vi "projet.vi"() -> ()   [LabVIEW 2020]
panel:
  out "message":string
  out "etage":i32
  out "A":bool
  out "E3":bool
  in  "C_3":bool
  in  "C_ 2":bool
  in  "C_1":bool
  in  "C_0":bool
  in  "3 Button":bool
  in  "2 Button":bool
  in  "1 Button":bool
  in  "0 Button":bool
  out "RDC":bool
  out "E1":bool
  out "E2":bool
  # "dans ce  projet :\nona 5 evenements :\n              -wait for postion (l'attente pour cliquer sur les buttons)\n             - le clique sur le button 0  (appel de l'ascenseur au RDC)\n              - le clique sur le button 1 (appel de l'ascenseur au  1ère étage)\n               -le clique sur le button 2  (appel de l'ascenseur au  2ème étage)\n              - le clique sur le button 3 (appel de l'ascenseur au  3ème étage)\n-un message  pour expliquer  la 1er etape de demarage de ce projet \n-chaque transition d' un etage à un  autre  se fait par le clique sur les capteur indiquant\nl'étage actuel et afficher son numéro dans l 'indicateur  \"etage\"\n-led A  : \"open\" lorsque  ona arrivee   à la destination \nona fait la comparison avec les button de capteur   dans chaque evenement \npar exemple  lorsque ona clique sur le button1 on peut trouver dans C-3 ,C-2,C-1,C-0\net la clique   sur le capteur C-3 va desactiver les capteur C-0 , C-1 et l' atttente pour cliquer\nsur le capteur C-2 , ce clique permet d'activer C-1et desactiverC-3  ect ..."
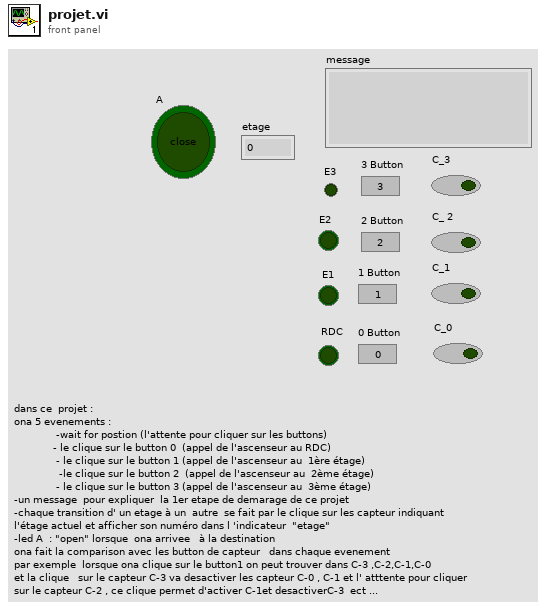
[diagram p1: front panel]
types:
  T1 = enum16{"wait for postion", "B1", "B2", "B3", "B0"}
  T2 = enum8{"Enabled", "Disabled", "Disabled and Grayed Out"}
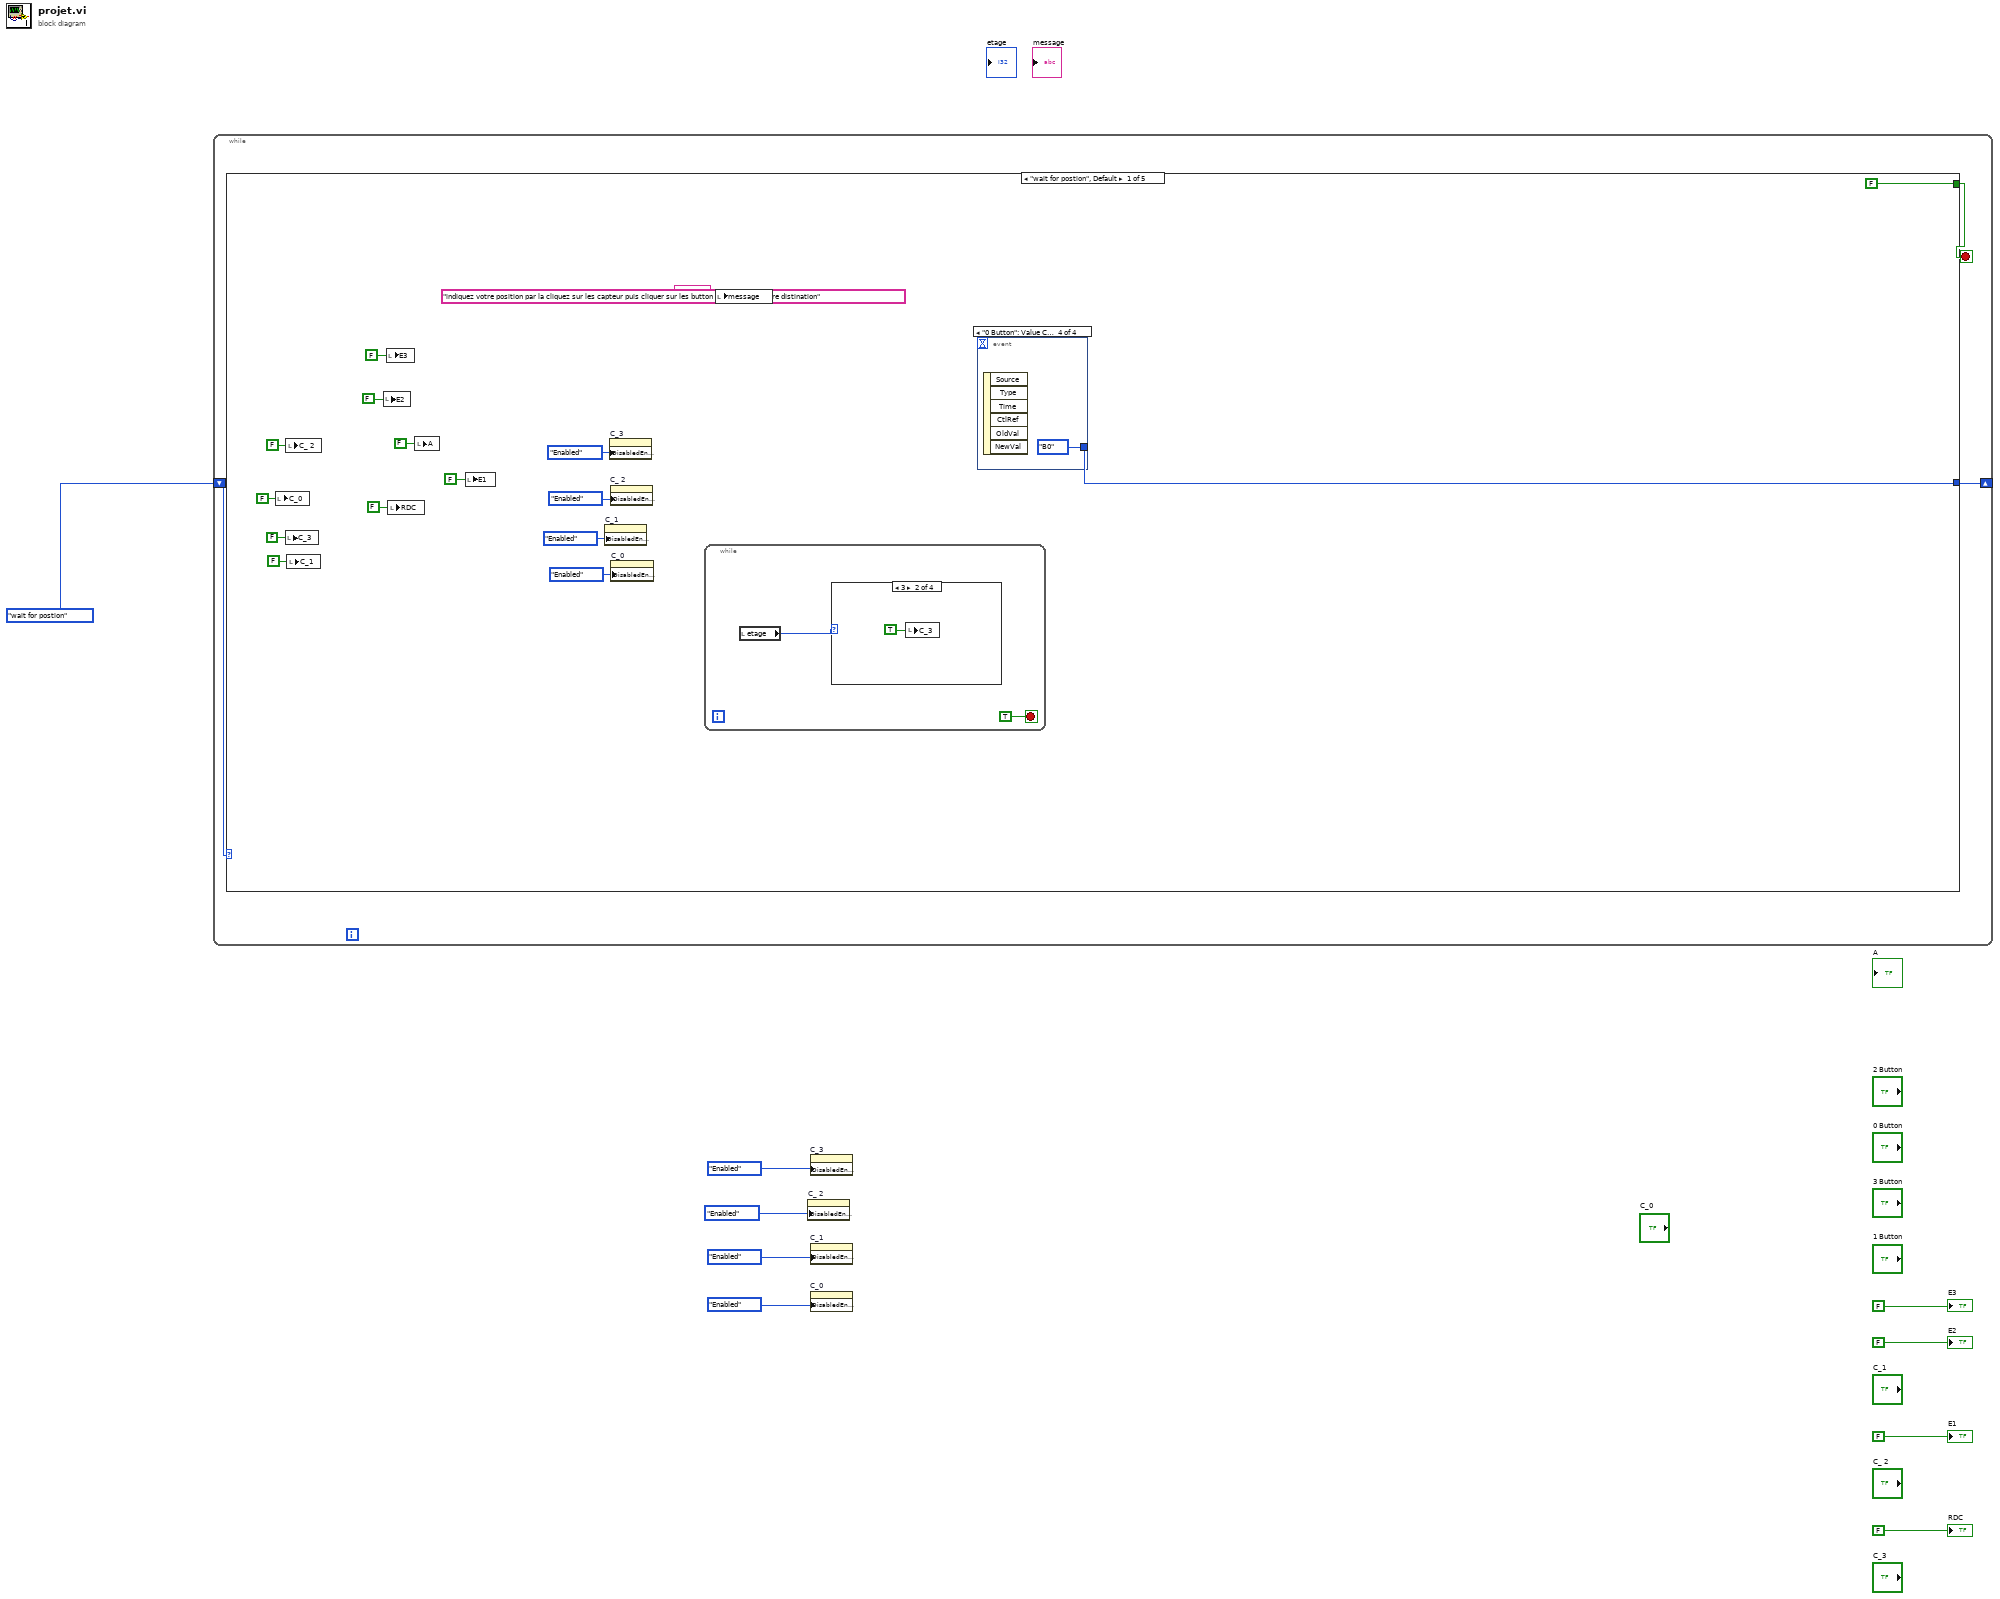
[diagram p0: block diagram]
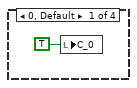
[diagram p2: hidden frame]
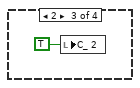
[diagram p3: hidden frame]
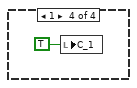
[diagram p4: hidden frame]
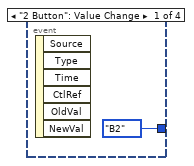
[diagram p5: hidden frame]
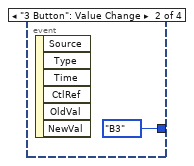
[diagram p6: hidden frame]
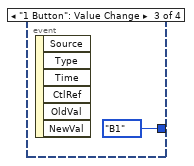
[diagram p7: hidden frame]
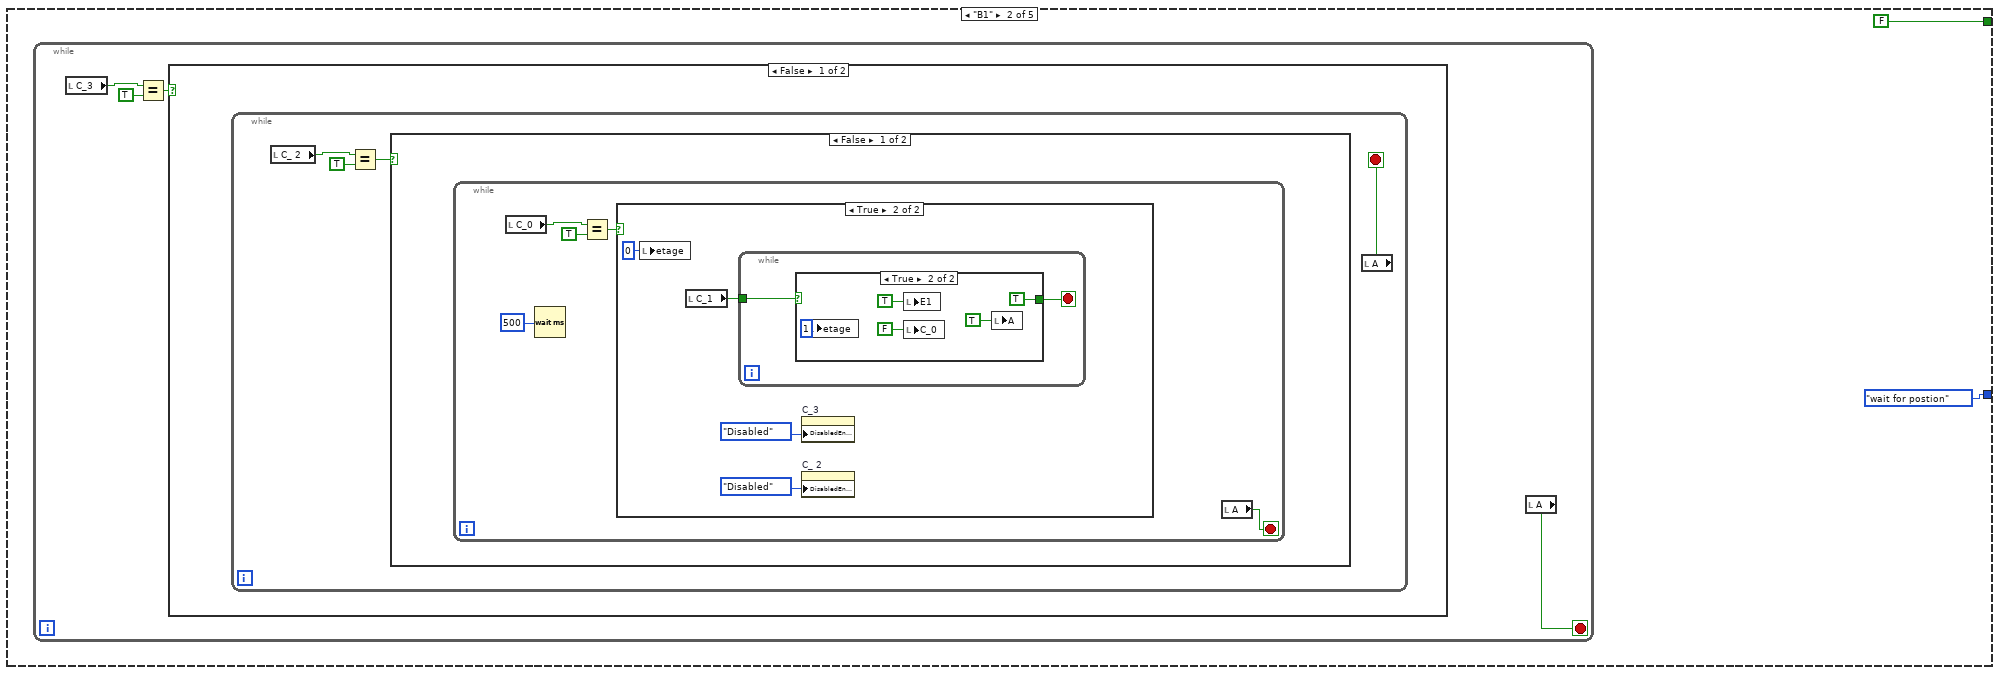
[diagram p8: hidden frame]
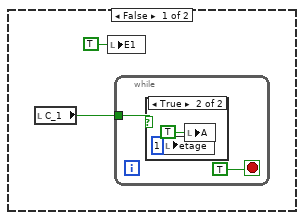
[diagram p9: hidden frame]
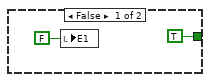
[diagram p11: hidden frame]
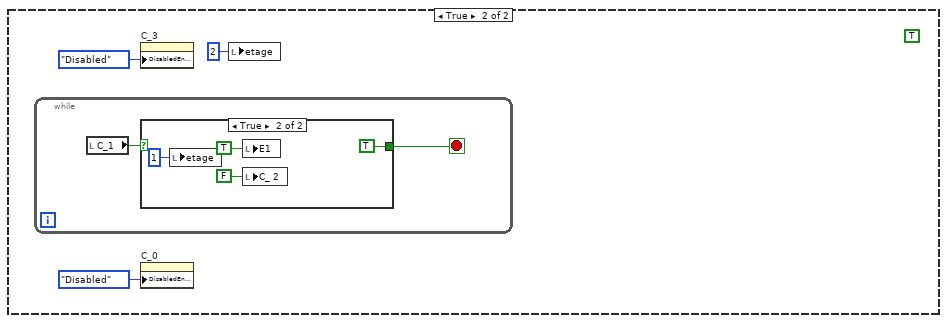
[diagram p12: hidden frame]
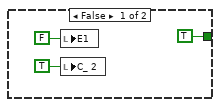
[diagram p13: hidden frame]
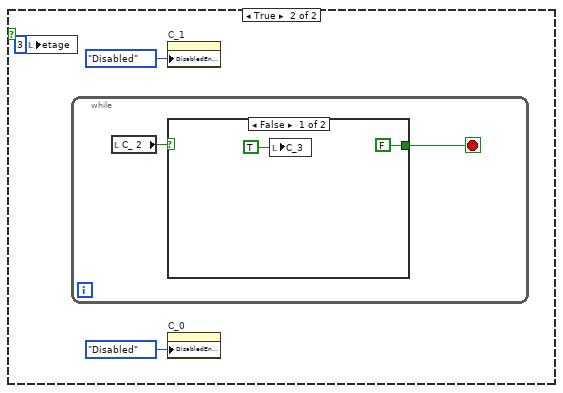
[diagram p14: hidden frame]
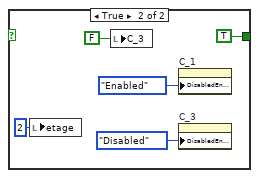
[diagram p15: hidden frame]
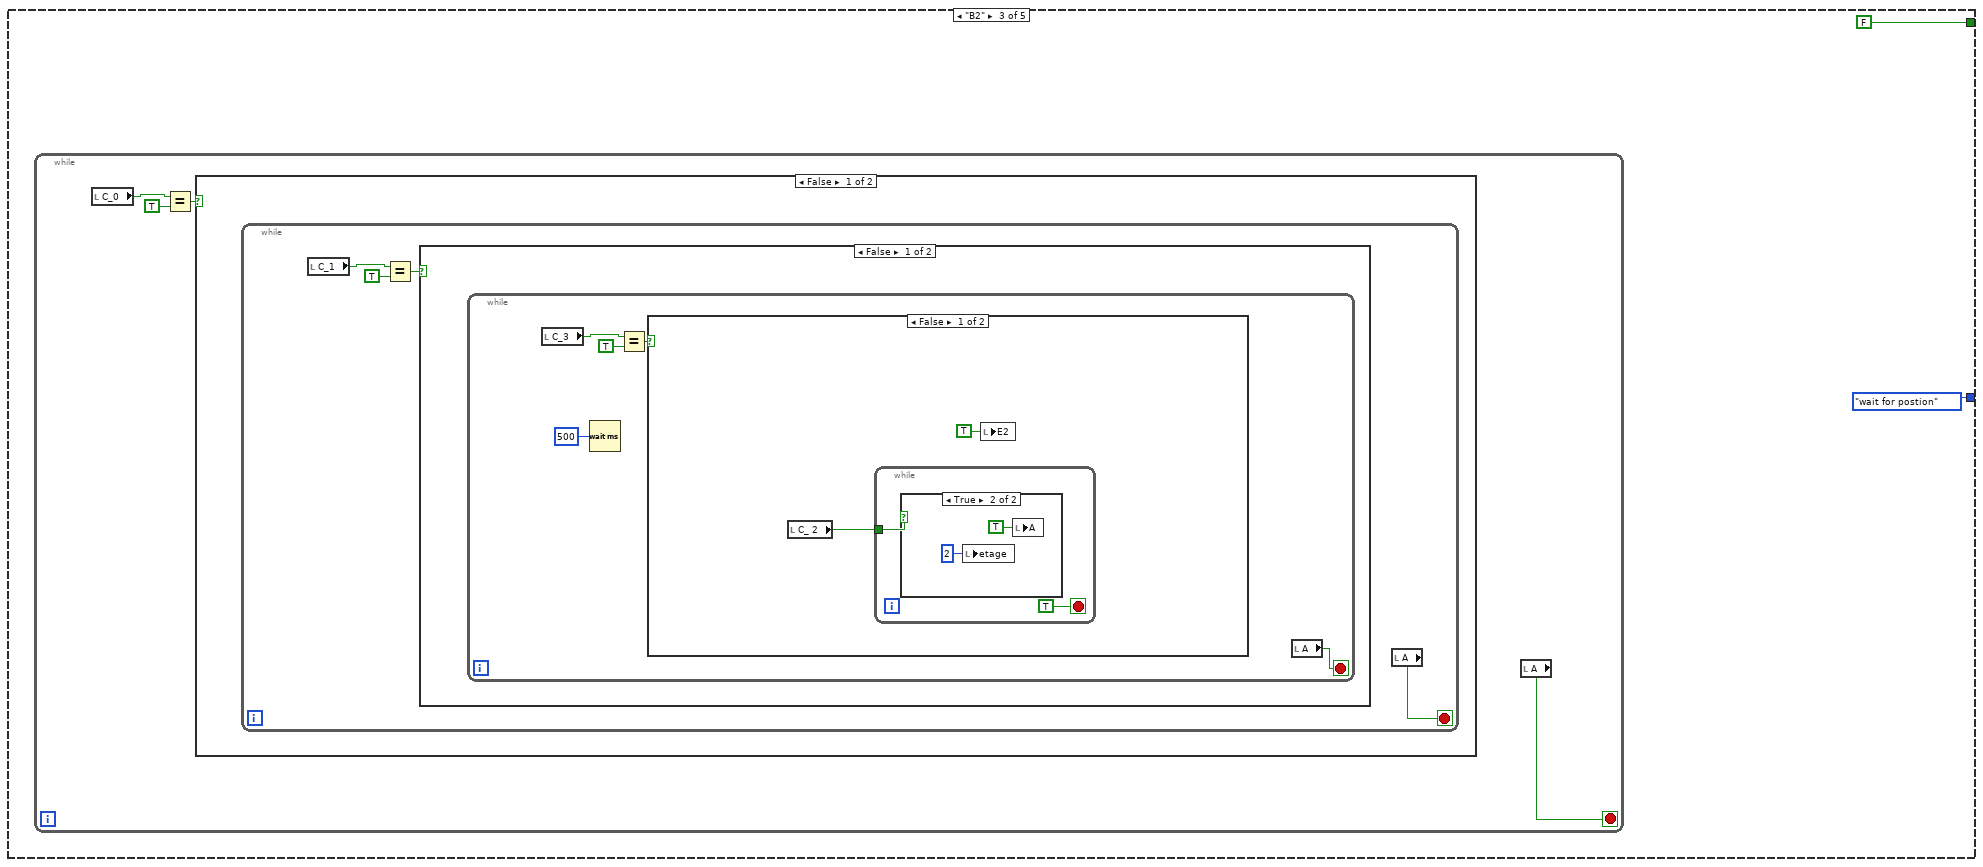
[diagram p16: hidden frame]
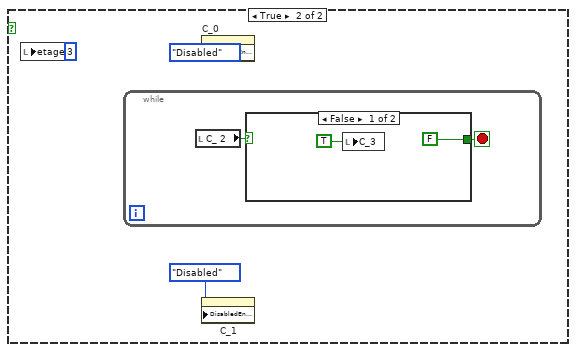
[diagram p18: hidden frame]
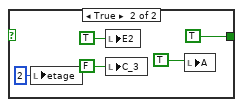
[diagram p19: hidden frame]
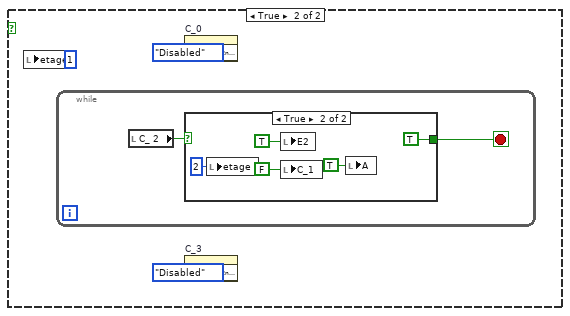
[diagram p20: hidden frame]
diagram:
  n1 = while {
    shift-right: [w11] -> _
    shift-left: T1."wait for postion" -> [w10]
    stop <- w12 stop-if-true
    n2 = case shown="\"wait for postion\", Default" w10 {
      tunnel: [w28 T1."wait for postion" T1."wait for postion" T1."wait for postion" T1."wait for postion"] -> w11
      tunnel: [FALSE FALSE FALSE FALSE FALSE] -> w12
      frame "wait for postion", Default {
        n3 = local write "C_0"(FALSE ("C_0")) -> ()
        n4 = local write "C_3"(FALSE ("C_3")) -> ()
        n5 = local write "C_ 2"(FALSE ("C_ 2")) -> ()
        n6 = local write "C_1"(FALSE ("C_1")) -> ()
        n7 = local write "E2"(FALSE ("E2")) -> ()
        n8 = local write "E3"(FALSE ("E3")) -> ()
        n9 = local write "RDC"(FALSE ("RDC")) -> ()
        n10 = local write "A"(FALSE ("A")) -> ()
        n11 = local write "E1"(FALSE ("E1")) -> ()
        n12 = property on="C_1" class="Bool (strict)"("DisabledEnum"=T2."Enabled" ("Disabled")) -> ()  [unwired: 2 in, 2 out]
        n13 = property on="C_3" class="Bool (strict)"("DisabledEnum"=T2."Enabled" ("Disabled")) -> ()  [unwired: 2 in, 2 out]
        n14 = property on="C_ 2" class="Bool (strict)"("DisabledEnum"=T2."Enabled" ("Disabled")) -> ()  [unwired: 2 in, 2 out]
        n15 = property on="C_0" class="Bool (strict)"("DisabledEnum"=T2."Enabled" ("Disabled")) -> ()  [unwired: 2 in, 2 out]
        n16 = while {
          stop <- TRUE stop-if-true
          n17 = local read "etage"() -> (w30:i32)
          n18 = case shown="3" w30 {
            frame 0, Default {
              n19 = local write "C_0"(TRUE ("C_0")) -> ()
            }
            frame 3 {
              n20 = local write "C_3"(TRUE ("C_3")) -> ()
            }
            frame 2 {
              n21 = local write "C_ 2"(TRUE ("C_ 2")) -> ()
            }
            frame 1 {
              n22 = local write "C_1"(TRUE ("C_1")) -> ()
            }
          }
        }
        n23 = local write "message"("indiquez votre position par la cliquez sur les capteur puis cliquer sur les button pour indiquer votre distination" ("message erreur")) -> ()
        n24 = event shown="[3] \"0 Button\": Value Change" {
          selector: _ -> [_ _ _ _]
          dyn-events: _ -> [_ _ _ _]
          timeout: _ -> [_ _ _ _]
          tunnel: [T1."B2" T1."B3" T1."B1" T1."B0"] -> w28
          event "2 Button": Value Change {
            n25 = event-data() -> ()  [unwired: 1 in, 6 out]
          }
          event "3 Button": Value Change {
            n26 = event-data() -> ()  [unwired: 1 in, 6 out]
          }
          event "1 Button": Value Change {
            n27 = event-data() -> ()  [unwired: 1 in, 6 out]
          }
          event "0 Button": Value Change {
            n28 = event-data() -> ()  [unwired: 1 in, 6 out]
          }
        }
      }
      frame "B1" {
        n29 = while {
          stop <- w41 stop-if-true
          n30 = local read "C_3"() -> (w44:bool)
          n31 = Equal?(x=w44, y=TRUE) -> (x = y?=w42:bool)
          n32 = case shown="False" w42 {
            frame False {
              n33 = while {
                stop <- w45 stop-if-true
                n34 = local read "C_ 2"() -> (w48:bool)
                n35 = Equal?(x=w48, y=TRUE) -> (x = y?=w46:bool)
                n36 = case shown="False" w46 {
                  frame False {
                    n37 = while {
                      stop <- w50 stop-if-true
                      n38 = local read "C_0"() -> (w53:bool)
                      n39 = Wait (ms)(milliseconds to wait=u32 500) -> ()  [unwired: 1 out]
                      n40 = Equal?(x=w53, y=TRUE) -> (x = y?=w51:bool)
                      n41 = case shown="True" w51 {
                        frame False {
                          n42 = local read "C_1"() -> (w54:bool)
                          n43 = local write "E1"(TRUE ("E1")) -> ()
                          n44 = while {
                            tunnel: w54 -> [w57]
                            stop <- TRUE stop-if-true
                            n45 = case shown="True" w57 {
                              frame False {
                              }
                              frame True {
                                n46 = local write "etage"(1 ("etage")) -> ()
                                n47 = local write "A"(TRUE ("A")) -> ()
                              }
                            }
                          }
                        }
                        frame True {
                          n48 = local write "etage"(0 ("etage")) -> ()
                          n49 = local read "C_1"() -> (w61:bool)
                          n50 = while {
                            tunnel: w61 -> [w65]
                            stop <- w64 stop-if-true
                            n51 = case shown="True" w65 {
                              tunnel: [TRUE TRUE] -> w64
                              frame False {
                                n52 = local write "E1"(FALSE ("E1")) -> ()
                              }
                              frame True {
                                n53 = local write "etage"(1 ("etage")) -> ()
                                n54 = local write "E1"(TRUE ("E1")) -> ()
                                n55 = local write "C_0"(FALSE ("C_0")) -> ()
                                n56 = local write "A"(TRUE ("Boolean")) -> ()
                              }
                            }
                          }
                          n57 = property on="C_3" class="Bool (strict)"("DisabledEnum"=T2."Disabled" ("Disabled")) -> ()  [unwired: 2 in, 2 out]
                          n58 = property on="C_ 2" class="Bool (strict)"("DisabledEnum"=T2."Disabled" ("Disabled")) -> ()  [unwired: 2 in, 2 out]
                        }
                      }
                      n59 = local read "A"() -> (w50:bool)
                    }
                  }
                  frame True {
                    (unwired) TRUE
                    n60 = while {
                      stop <- w76 stop-if-true
                      n61 = local read "C_1"() -> (w77:bool)
                      n62 = case shown="True" w77 {
                        tunnel: [TRUE TRUE] -> w76
                        frame False {
                          n63 = local write "E1"(FALSE ("E1")) -> ()
                          n64 = local write "C_ 2"(TRUE ("C_ 2")) -> ()
                        }
                        frame True {
                          n65 = local write "etage"(1 ("etage")) -> ()
                          n66 = local write "E1"(TRUE ("error")) -> ()
                          n67 = local write "C_ 2"(FALSE ("C_ 2")) -> ()
                        }
                      }
                    }
                    n68 = property on="C_3" class="Bool (strict)"("DisabledEnum"=T2."Disabled" ("Disabled")) -> ()  [unwired: 2 in, 2 out]
                    n69 = property on="C_0" class="Bool (strict)"("DisabledEnum"=T2."Disabled" ("Disabled")) -> ()  [unwired: 2 in, 2 out]
                    n70 = local write "etage"(2 ("etage")) -> ()
                  }
                }
                n71 = local read "A"() -> (w45:bool)
              }
            }
            frame True {
              n72 = local write "etage"(3 ("etage")) -> ()
              n73 = while {
                stop <- w88 stop-if-true
                n74 = local read "C_ 2"() -> (w89:bool)
                n75 = case shown="False" w89 {
                  tunnel: [FALSE TRUE] -> w88
                  frame False {
                    n76 = local write "C_3"(TRUE ("E1 2")) -> ()
                  }
                  frame True {
                    n77 = local write "etage"(2 ("etage")) -> ()
                    n78 = local write "C_3"(FALSE ("RDC 2")) -> ()
                    n79 = property on="C_1" class="Bool (strict)"("DisabledEnum"=T2."Enabled" ("Disabled")) -> ()  [unwired: 2 in, 2 out]
                    n80 = property on="C_3" class="Bool (strict)"("DisabledEnum"=T2."Disabled" ("Disabled")) -> ()  [unwired: 2 in, 2 out]
                  }
                }
              }
              n81 = property on="C_1" class="Bool (strict)"("DisabledEnum"=T2."Disabled" ("Disabled")) -> ()  [unwired: 2 in, 2 out]
              n82 = property on="C_0" class="Bool (strict)"("DisabledEnum"=T2."Disabled" ("Disabled")) -> ()  [unwired: 2 in, 2 out]
            }
          }
          n83 = local read "A"() -> (w41:bool)
        }
      }
      frame "B2" {
        n84 = while {
          stop <- w99 stop-if-true
          n85 = local read "C_0"() -> (w102:bool)
          n86 = Equal?(x=w102, y=TRUE) -> (x = y?=w100:bool)
          n87 = case shown="False" w100 {
            frame False {
              n88 = while {
                stop <- w103 stop-if-true
                n89 = local read "C_1"() -> (w106:bool)
                n90 = Equal?(x=w106, y=TRUE) -> (x = y?=w104:bool)
                n91 = case shown="False" w104 {
                  frame False {
                    n92 = while {
                      stop <- w108 stop-if-true
                      n93 = local read "C_3"() -> (w111:bool)
                      n94 = Wait (ms)(milliseconds to wait=u32 500) -> ()  [unwired: 1 out]
                      n95 = Equal?(x=w111, y=TRUE) -> (x = y?=w109:bool)
                      n96 = case shown="False" w109 {
                        frame False {
                          n97 = local read "C_ 2"() -> (w112:bool)
                          n98 = while {
                            tunnel: w112 -> [w115]
                            stop <- TRUE stop-if-true
                            n99 = case shown="True" w115 {
                              frame False {
                              }
                              frame True {
                                n100 = local write "etage"(2 ("etage")) -> ()
                                n101 = local write "A"(TRUE ("A")) -> ()
                              }
                            }
                          }
                          n102 = local write "E2"(TRUE ("E2")) -> ()
                        }
                        frame True {
                          n103 = local write "etage"(3 ("etage")) -> ()
                          n104 = while {
                            stop <- w121 stop-if-true
                            n105 = local read "C_ 2"() -> (w122:bool)
                            n106 = case shown="False" w122 {
                              tunnel: [FALSE TRUE] -> w121
                              frame False {
                                n107 = local write "C_3"(TRUE ("E2 2")) -> ()
                              }
                              frame True {
                                n108 = local write "etage"(2 ("etage")) -> ()
                                n109 = local write "E2"(TRUE ("E2 2")) -> ()
                                n110 = local write "C_3"(FALSE ("E1 2")) -> ()
                                n111 = local write "A"(TRUE ("Boolean")) -> ()
                              }
                            }
                          }
                          n112 = property on="C_0" class="Bool (strict)"("DisabledEnum"=T2."Disabled" ("Disabled")) -> ()  [unwired: 2 in, 2 out]
                          n113 = property on="C_1" class="Bool (strict)"("DisabledEnum"=T2."Disabled" ("Disabled")) -> ()  [unwired: 2 in, 2 out]
                        }
                      }
                      n114 = local read "A"() -> (w108:bool)
                    }
                  }
                  frame True {
                    n115 = local write "etage"(1 ("etage")) -> ()
                    n116 = while {
                      stop <- w133 stop-if-true
                      n117 = local read "C_ 2"() -> (w134:bool)
                      n118 = case shown="True" w134 {
                        tunnel: [FALSE TRUE] -> w133
                        frame False {
                          n119 = local write "C_1"(TRUE ("E1 2")) -> ()
                          n120 = local write "E2"(FALSE ("E2")) -> ()
                        }
                        frame True {
                          n121 = local write "etage"(2 ("etage")) -> ()
                          n122 = local write "E2"(TRUE ("E1 2")) -> ()
                          n123 = local write "C_1"(FALSE ("RDC 2")) -> ()
                          n124 = local write "A"(TRUE ("A")) -> ()
                        }
                      }
                    }
                    n125 = property on="C_0" class="Bool (strict)"("DisabledEnum"=T2."Disabled" ("Disabled")) -> ()  [unwired: 2 in, 2 out]
                    n126 = property on="C_3" class="Bool (strict)"("DisabledEnum"=T2."Disabled" ("Disabled")) -> ()  [unwired: 2 in, 2 out]
                  }
                }
                n127 = local read "A"() -> (w103:bool)
              }
            }
            frame True {
              n128 = local write "etage"(0 ("etage")) -> ()
              n129 = while {
                stop <- w146 stop-if-true
                n130 = local read "C_1"() -> (w147:bool)
                n131 = case shown="True" w147 {
                  tunnel: [TRUE TRUE] -> w146
                  frame False {
                    n132 = local write "C_0"(TRUE ("E2 2")) -> ()
                  }
                  frame True {
                    n133 = local write "etage"(1 ("etage")) -> ()
                    n134 = local write "C_0"(FALSE ("E3 2")) -> ()
                    n135 = property on="C_ 2" class="Bool (strict)"("DisabledEnum"=T2."Enabled" ("Disabled")) -> ()  [unwired: 2 in, 2 out]
                  }
                }
              }
              n136 = property on="C_ 2" class="Bool (strict)"("DisabledEnum"=T2."Disabled" ("Disabled")) -> ()  [unwired: 2 in, 2 out]
              n137 = property on="C_3" class="Bool (strict)"("DisabledEnum"=T2."Disabled" ("Disabled")) -> ()  [unwired: 2 in, 2 out]
            }
          }
          n138 = local read "A"() -> (w99:bool)
        }
      }
      frame "B3" {
        n139 = while {
          stop <- w156 stop-if-true
          n140 = local read "C_0"() -> (w159:bool)
          n141 = Equal?(x=w159, y=TRUE) -> (x = y?=w157:bool)
          n142 = case shown="True" w157 {
            frame False {
              n143 = while {
                stop <- w160 stop-if-true
                n144 = local read "C_1"() -> (w163:bool)
                n145 = Equal?(x=w163, y=TRUE) -> (x = y?=w161:bool)
                n146 = case shown="False" w161 {
                  frame False {
                    n147 = while {
                      stop <- w165 stop-if-true
                      n148 = Wait (ms)(milliseconds to wait=u32 500) -> ()  [unwired: 1 out]
                      n149 = local read "C_ 2"() -> (w168:bool)
                      n150 = Equal?(x=w168, y=TRUE) -> (x = y?=w166:bool)
                      n151 = case shown="False" w166 {
                        frame False {
                          n152 = local write "E3"(TRUE ("E3")) -> ()
                          n153 = local read "C_3"() -> (w169:bool)
                          n154 = while {
                            tunnel: w169 -> [w172]
                            stop <- TRUE stop-if-true
                            n155 = case shown="True" w172 {
                              frame False {
                              }
                              frame True {
                                n156 = local write "etage"(3 ("etage")) -> ()
                                n157 = local write "A"(TRUE ("A")) -> ()
                              }
                            }
                          }
                        }
                        frame True {
                          n158 = local write "etage"(2 ("etage")) -> ()
                          n159 = while {
                            stop <- w178 stop-if-true
                            n160 = local read "C_3"() -> (w179:bool)
                            n161 = case shown="True" w179 {
                              tunnel: [FALSE TRUE] -> w178
                              frame False {
                                n162 = local write "E3"(FALSE ("E3 2")) -> ()
                              }
                              frame True {
                                n163 = local write "etage"(3 ("etage")) -> ()
                                n164 = local write "E3"(TRUE ("E3 2")) -> ()
                                n165 = local write "C_ 2"(FALSE ("E2 2")) -> ()
                                n166 = property on="C_ 2" class="Bool (strict)"("DisabledEnum"=T2."Enabled" ("Disabled")) -> ()  [unwired: 2 in, 2 out]
                                n167 = local write "A"(TRUE ("Boolean")) -> ()
                              }
                            }
                          }
                          n168 = property on="C_1" class="Bool (strict)"("DisabledEnum"=T2."Disabled" ("Disabled")) -> ()  [unwired: 2 in, 2 out]
                          n169 = property on="C_0" class="Bool (strict)"("DisabledEnum"=T2."Disabled" ("Disabled")) -> ()  [unwired: 2 in, 2 out]
                        }
                      }
                      n170 = local read "A"() -> (w165:bool)
                    }
                  }
                  frame True {
                    n171 = while {
                      stop <- w191 stop-if-true
                      n172 = local read "C_ 2"() -> (w192:bool)
                      n173 = case shown="True" w192 {
                        tunnel: [FALSE TRUE] -> w191
                        frame False {
                          n174 = local write "C_1"(TRUE ("E2 2")) -> ()
                        }
                        frame True {
                          n175 = local write "etage"(2 ("etage")) -> ()
                          n176 = local write "C_1"(FALSE ("E1 2")) -> ()
                          n177 = property on="C_1" class="Bool (strict)"("DisabledEnum"=T2."Disabled" ("Disabled")) -> ()  [unwired: 2 in, 2 out]
                          n178 = property on="C_3" class="Bool (strict)"("DisabledEnum"=T2."Enabled" ("Disabled")) -> ()  [unwired: 2 in, 2 out]
                        }
                      }
                    }
                    n179 = property on="C_0" class="Bool (strict)"("DisabledEnum"=T2."Disabled" ("Disabled")) -> ()  [unwired: 2 in, 2 out]
                    n180 = property on="C_3" class="Bool (strict)"("DisabledEnum"=T2."Disabled" ("Disabled")) -> ()  [unwired: 2 in, 2 out]
                    n181 = local write "etage"(1 ("etage")) -> ()
                  }
                }
                n182 = local read "A"() -> (w160:bool)
              }
            }
            frame True {
              n183 = local write "etage"(0 ("etage")) -> ()
              n184 = while {
                stop <- w203 stop-if-true
                n185 = local read "C_1"() -> (w204:bool)
                n186 = case shown="False" w204 {
                  tunnel: [FALSE TRUE] -> w203
                  frame False {
                    n187 = local write "C_0"(TRUE ("E1 2")) -> ()
                  }
                  frame True {
                    n188 = local write "etage"(1 ("etage")) -> ()
                    n189 = local write "C_0"(FALSE ("RDC 2")) -> ()
                    n190 = property on="C_ 2" class="Bool (strict)"("DisabledEnum"=T2."Enabled" ("Disabled")) -> ()  [unwired: 2 in, 2 out]
                    n191 = property on="C_0" class="Bool (strict)"("DisabledEnum"=T2."Disabled" ("Disabled")) -> ()  [unwired: 2 in, 2 out]
                  }
                }
              }
              n192 = property on="C_3" class="Bool (strict)"("DisabledEnum"=T2."Disabled" ("Disabled")) -> ()  [unwired: 2 in, 2 out]
              n193 = property on="C_ 2" class="Bool (strict)"("DisabledEnum"=T2."Disabled" ("Disabled")) -> ()  [unwired: 2 in, 2 out]
            }
          }
          n194 = local read "A"() -> (w156:bool)
        }
      }
      frame "B0" {
        n195 = while {
          stop <- w214 stop-if-true
          n196 = local read "C_3"() -> (w217:bool)
          n197 = Equal?(x=w217, y=TRUE) -> (x = y?=w215:bool)
          n198 = case shown="False" w215 {
            frame False {
              n199 = while {
                stop <- w218 stop-if-true
                n200 = local read "C_ 2"() -> (w221:bool)
                n201 = Equal?(x=w221, y=TRUE ("x")) -> (x = y?=w219:bool)
                n202 = case shown="False" w219 {
                  frame False {
                    n203 = while {
                      stop <- w222 stop-if-true
                      n204 = local read "C_1"() -> (w226:bool)
                      n205 = Wait (ms)(milliseconds to wait=u32 500) -> ()  [unwired: 1 out]
                      n206 = Equal?(x=w226, y=TRUE) -> (x = y?=w224:bool)
                      n207 = case shown="False" w224 {
                        frame False {
                          n208 = local read "C_0"() -> (w227:bool)
                          n209 = local write "RDC"(TRUE ("RDC")) -> ()
                          n210 = while {
                            tunnel: w227 -> [w230]
                            stop <- TRUE stop-if-true
                            n211 = case shown="True" w230 {
                              frame False {
                              }
                              frame True {
                                n212 = local write "etage"(0 ("etage")) -> ()
                                n213 = local write "A"(TRUE ("A")) -> ()
                              }
                            }
                          }
                        }
                        frame True {
                          n214 = local write "etage"(1 ("etage")) -> ()
                          n215 = while {
                            stop <- w236 stop-if-true
                            n216 = local read "C_0"() -> (w237:bool)
                            n217 = case shown="True" w237 {
                              tunnel: [FALSE TRUE] -> w236
                              frame False {
                                n218 = local write "RDC"(FALSE ("RDC 2")) -> ()
                              }
                              frame True {
                                n219 = local write "etage"(1 ("etage")) -> ()
                                n220 = local write "RDC"(TRUE ("RDC 2")) -> ()
                                n221 = local write "C_1"(FALSE ("C_1")) -> ()
                                n222 = property on="C_1" class="Bool (strict)"("DisabledEnum"=T2."Disabled" ("Disabled")) -> ()  [unwired: 2 in, 2 out]
                                n223 = local write "A"(TRUE ("Boolean")) -> ()
                              }
                            }
                          }
                          n224 = property on="C_ 2" class="Bool (strict)"("DisabledEnum"=T2."Disabled" ("Disabled")) -> ()  [unwired: 2 in, 2 out]
                          n225 = property on="C_3" class="Bool (strict)"("DisabledEnum"=T2."Disabled" ("Disabled")) -> ()  [unwired: 2 in, 2 out]
                        }
                      }
                      n226 = local read "A"() -> (w222:bool)
                    }
                  }
                  frame True {
                    n227 = while {
                      stop <- w249 stop-if-true
                      n228 = local read "C_1"() -> (w250:bool)
                      n229 = case shown="True" w250 {
                        tunnel: [FALSE TRUE] -> w249
                        frame False {
                          n230 = local write "C_ 2"(TRUE ("E1 2")) -> ()
                        }
                        frame True {
                          n231 = local write "etage"(1 ("etage")) -> ()
                          n232 = local write "C_ 2"(FALSE ("E2 2")) -> ()
                          n233 = property on="C_0" class="Bool (strict)"("DisabledEnum"=T2."Enabled" ("Disabled")) -> ()  [unwired: 2 in, 2 out]
                        }
                      }
                    }
                    n234 = property on="C_3" class="Bool (strict)"("DisabledEnum"=T2."Disabled" ("Disabled")) -> ()  [unwired: 2 in, 2 out]
                    n235 = property on="C_0" class="Bool (strict)"("DisabledEnum"=T2."Disabled" ("Disabled")) -> ()  [unwired: 2 in, 2 out]
                    n236 = local write "etage"(2 ("etage")) -> ()
                  }
                }
                n237 = local read "A"() -> (w218:bool)
              }
            }
            frame True {
              n238 = local write "etage"(3 ("etage")) -> ()
              n239 = while {
                stop <- w259 stop-if-true
                n240 = local read "C_ 2"() -> (w260:bool)
                n241 = Wait (ms)(milliseconds to wait=u32 500) -> ()  [unwired: 1 out]
                n242 = case shown="True" w260 {
                  tunnel: [FALSE TRUE] -> w259
                  frame False {
                    n243 = local write "C_3"(TRUE ("E3 2")) -> ()
                  }
                  frame True {
                    n244 = local write "etage"(2 ("etage")) -> ()
                    n245 = local write "C_3"(FALSE ("E2 2")) -> ()
                    n246 = property on="C_1" class="Bool (strict)"("DisabledEnum"=T2."Enabled" ("Disabled")) -> ()  [unwired: 2 in, 2 out]
                  }
                }
              }
            }
          }
          n247 = local read "A"() -> (w214:bool)
        }
      }
    }
  }
  n248 = property on="C_ 2" class="Bool (strict)"("DisabledEnum"=T2."Enabled" ("Disabled")) -> ()  [unwired: 2 in, 2 out]
  n249 = property on="C_3" class="Bool (strict)"("DisabledEnum"=T2."Enabled" ("Disabled")) -> ()  [unwired: 2 in, 2 out]
  n250 = property on="C_1" class="Bool (strict)"("DisabledEnum"=T2."Enabled" ("Disabled")) -> ()  [unwired: 2 in, 2 out]
  n251 = property on="C_0" class="Bool (strict)"("DisabledEnum"=T2."Enabled" ("Disabled")) -> ()  [unwired: 2 in, 2 out]
  "E2" <- FALSE ("E2")
  "E1" <- FALSE ("E1")
  "RDC" <- FALSE ("RDC")
  "E3" <- FALSE ("E3")
